vi "set user path.vi"(8 "error in (no error)":errorcluster, 10 "User VI Path":path) -> (0 "error out":errorcluster)   [LabVIEW 2013]
panel:
  out "User VI Path 2":path
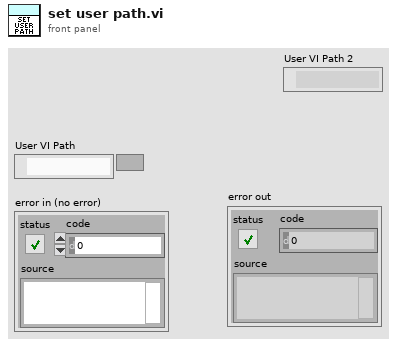
[diagram p1: front panel]
types:
  T1 = enum16{"open", "replace", "create", "open or create", "replace or create", "replace or create with confirmation"}
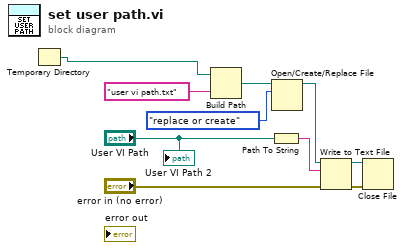
[diagram p0: block diagram]
diagram:
  n1 = Temporary Directory() -> (w1:path)
  n2 = Build Path(base path=w1, name or relative path="user vi path.txt") -> (appended path=w4:path)
  n3 = Path To String(path="User VI Path") -> (string=w7:string)
  n4 = Open/Create/Replace File(file path (use dialog)=w4, operation (0:open)=T1."replace or create") -> (refnum out=w2:refnum<file>)  [unwired: 4 in, 2 out]
  n5 = Write to Text File(file (use dialog)=w2, text=w7, error in="error in (no error)") -> (refnum out=w10:refnum<file>, error out=w9:errorcluster)  [unwired: 1 in, 1 out]
  n6 = Close File(refnum=w10, error in=w9) -> ()  [unwired: 2 out]
  "User VI Path 2" <- "User VI Path"
